vi "StringInputKeyboardSimulation_Tests.vi"(11 "error in (no error)":errorcluster) -> (15 "error out":errorcluster)   [LabVIEW 2016, in "DronaTest.lvlib"]
uses:
  DronaTest.lvlib
  APIs/Stimulus/KeyBoardSimulation/KeyboardSimulationForStringInput.vi
  APIs/Assert/AssertControlValue/Equal.vi
  <vilib>/addons/_JKI Toolkits/Caraya/classes/Test/Test.lvclass
  Drona.lvlib
  APIs/Assert/AssertControlValue/AssertControlValue.lvlib
  APIs/Stimulus/KeyBoardSimulation/KeyboardSimulation.lvlib
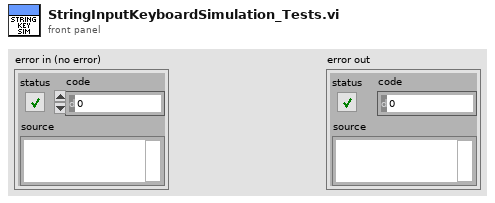
[diagram p1: front panel]
types:
  T1 = enum16{"Type all possible letters in keyboard", "TypeNegative25_ControlValueShouldBeNegative25", "Type255_ControlValueCoerceTo100", "TypeNegative257_ControlValueCoerceToNegative100"}[]
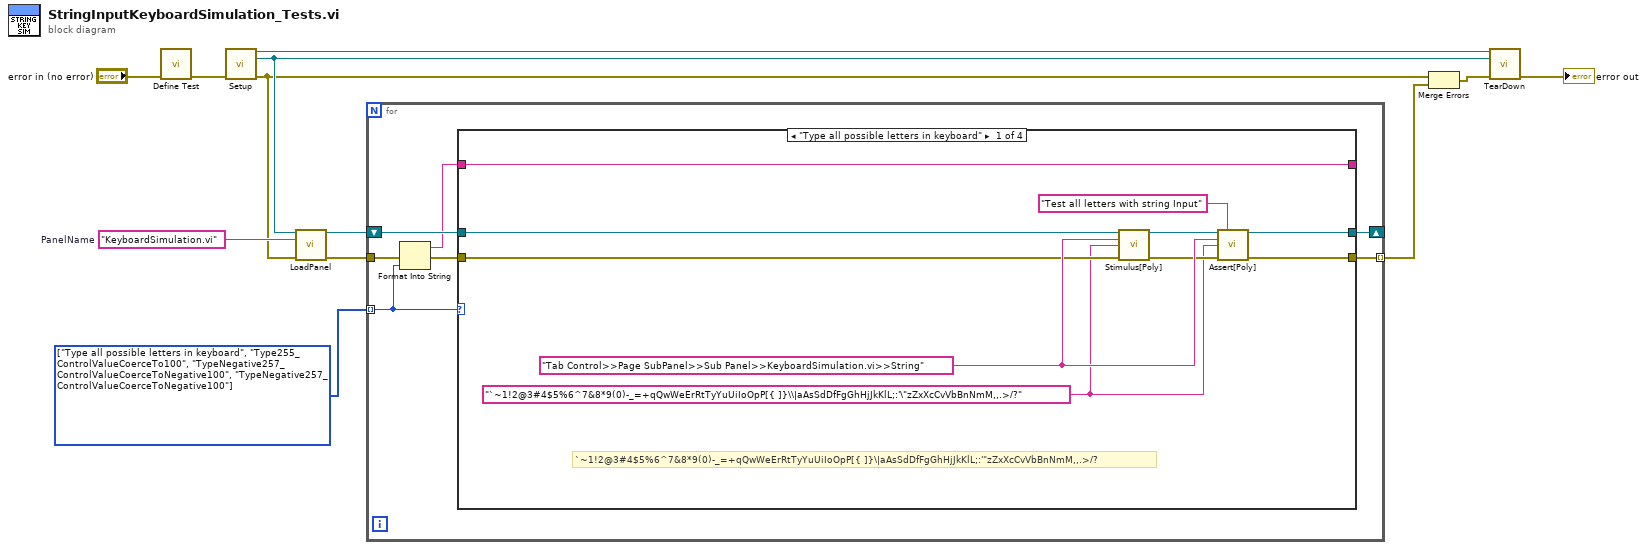
[diagram p0: block diagram]
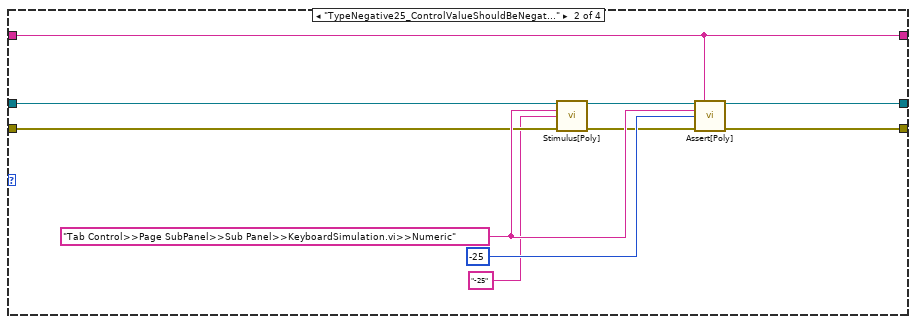
[diagram p2: hidden frame]
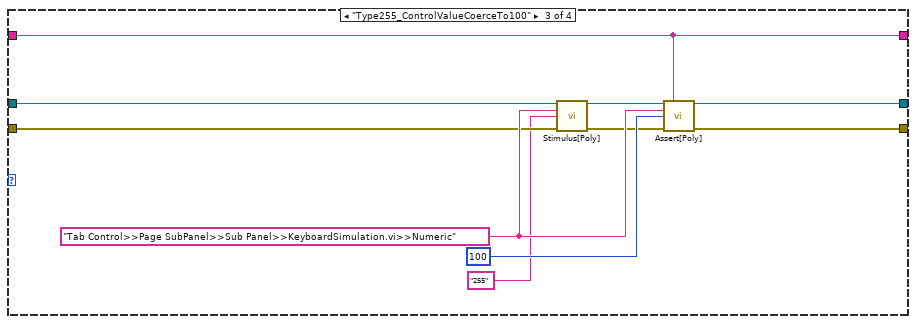
[diagram p3: hidden frame]
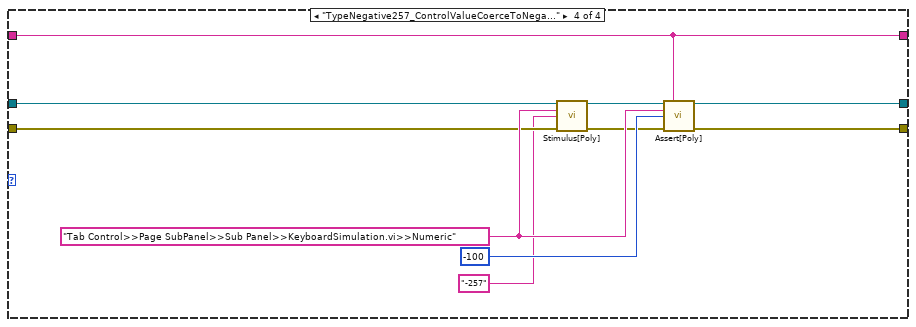
[diagram p4: hidden frame]
diagram:
  w10 = T1 [enum."Type all possible letters in keyboard", enum."Type255_ControlValueCoerceTo100", enum."TypeNegative257_ControlValueCoerceToNegative100", enum."TypeNegative257_ControlValueCoerceToNegative100"] items=["Type all possible letters in keyboard", "TypeNegative25_ControlValueShouldBeNegative25", "Type255_ControlValueCoerceTo100", "TypeNegative257_ControlValueCoerceToNegative100"] ("TestCases")
  w11 = "KeyboardSimulation.vi"  # PanelName
  n1 = call <vilib>:"Define Test.vi"("error in (no error)"="error in (no error)") -> ("error out"=w6:errorcluster)  [unwired: 9 in, 1 out]
  n2 = call "Setup.vi"("error in (no error)"=w6) -> ("Application Ref"=w3:refnum<vi>, "VI out"=w2:refnum<vi>, "error out"=w1:errorcluster)  [unwired: 12 in]
  n3 = call "LoadPanel.vi"("VI in"=w2, "Item Name"=w11, "error in (no error)"=w1) -> ("VI out"=w7:refnum<vi>, "error out"=w9:errorcluster)  [unwired: 11 in]
  n4 = for {
    tunnel: w10 -> [w14] mode=indexing
    shift-right: [w18] -> _
    shift-left: w7 -> [w19]
    tunnel: w9 -> [w17]
    tunnel: [w16] -> w8 mode=indexing
    n5 = Format Into String(error in=w17, w14) -> (resulting string=w13:string, error out=w15:errorcluster)  [unwired: 2 in]
    n6 = case shown="\"Type all possible letters in keyboard\"" w14 {
      tunnel: [w26 w35 w45 w55] -> w16
      tunnel: w19 -> [w25 w33 w43 w53]
      tunnel: [w24 w34 w44 w54] -> w18
      tunnel: w15 -> [w23 w32 w42 w52]
      tunnel: [w22 w31 w41 w51] -> _
      tunnel: w13 -> [w22 w31 w41 w51]
      frame "Type all possible letters in keyboard" {
        w20 = "`~1!2@3#4$5%6^7&8*9(0)-_=+qQwWeErRtTyYuUiIoOpP[{ ]}\\|aAsSdDfFgGhHjJkKlL;:'\"zZxXcCvVbBnNmM,,.>/?" ("Control Path")
        w29 = "Tab Control>>Page SubPanel>>Sub Panel>>KeyboardSimulation.vi>>String" ("Control Path")
        # "`~1!2@3#4$5%6^7&8*9(0)-_=+qQwWeErRtTyYuUiIoOpP[{ ]}\\|aAsSdDfFgGhHjJkKlL;:'\"zZxXcCvVbBnNmM,,.>/?"
        n7 = call-poly "Stimulus[Poly].vi"("VI Reference In"=w25, "Control Path"=w29, "String Value"=w20, "Error In"=w23) -> ("VI Reference Out"=w28:refnum<vi>, "Error Out"=w27:errorcluster)  [unwired: 10 in]
        n8 = call-poly "Assert[Poly].vi"("VI Reference In"=w28, "Test Label"="Test all letters with string Input", "Control Path"=w29, "Control Value"=w20, "Error In"=w27) -> ("VI Reference Out"=w24:refnum<vi>, "Error Out"=w26:errorcluster)  [unwired: 8 in, 1 out]
      }
      frame "TypeNegative25_ControlValueShouldBeNegative25" {
        w38 = "Tab Control>>Page SubPanel>>Sub Panel>>KeyboardSimulation.vi>>Numeric" ("Control Path")
        n9 = call-poly "Stimulus[Poly].vi"("VI Reference In"=w33, "Control Path"=w38, "String Value"="-25" ("string"), "Error In"=w32) -> ("VI Reference Out"=w36:refnum<vi>, "Error Out"=w37:errorcluster)  [unwired: 10 in]
        n10 = call-poly "Assert[Poly].vi"("VI Reference In"=w36, "Test Label"=w31, "Control Path"=w38, "Control Value"=-25 ("Control Path"), "Error In"=w37) -> ("VI Reference Out"=w34:refnum<vi>, "Error Out"=w35:errorcluster)  [unwired: 8 in, 1 out]
      }
      frame "Type255_ControlValueCoerceTo100" {
        w48 = "Tab Control>>Page SubPanel>>Sub Panel>>KeyboardSimulation.vi>>Numeric" ("Control Path")
        n11 = call-poly "Stimulus[Poly].vi"("VI Reference In"=w43, "Control Path"=w48, "String Value"="255" ("string"), "Error In"=w42) -> ("VI Reference Out"=w46:refnum<vi>, "Error Out"=w47:errorcluster)  [unwired: 10 in]
        n12 = call-poly "Assert[Poly].vi"("VI Reference In"=w46, "Test Label"=w41, "Control Path"=w48, "Control Value"=100 ("Control Path"), "Error In"=w47) -> ("VI Reference Out"=w44:refnum<vi>, "Error Out"=w45:errorcluster)  [unwired: 8 in, 1 out]
      }
      frame "TypeNegative257_ControlValueCoerceToNegative100" {
        w58 = "Tab Control>>Page SubPanel>>Sub Panel>>KeyboardSimulation.vi>>Numeric" ("Control Path")
        n13 = call-poly "Stimulus[Poly].vi"("VI Reference In"=w53, "Control Path"=w58, "String Value"="-257" ("string"), "Error In"=w52) -> ("VI Reference Out"=w56:refnum<vi>, "Error Out"=w57:errorcluster)  [unwired: 10 in]
        n14 = call-poly "Assert[Poly].vi"("VI Reference In"=w56, "Test Label"=w51, "Control Path"=w58, "Control Value"=-100 ("Control Path"), "Error In"=w57) -> ("VI Reference Out"=w54:refnum<vi>, "Error Out"=w55:errorcluster)  [unwired: 8 in, 1 out]
      }
    }
  }
  n15 = Merge Errors(w1, w8) -> (w5:errorcluster)
  n16 = call "TearDown.vi"("Application Ref"=w3, "VI in"=w2, "error in (no error)"=w5) -> ("error out"=→"error out":errorcluster)  [unwired: 12 in]
